vi "Memory.Pointer.Truncate U64.vi"(11 "U64":u64) -> (3 "truncated U64":u64)   [LabVIEW 2016, in "LabVIEW Memory Manager.lvlib" / "Memory.Pointer.lvclass"]
uses:
  Memory.Pointer.lvclass
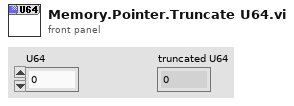
[diagram p1: front panel]
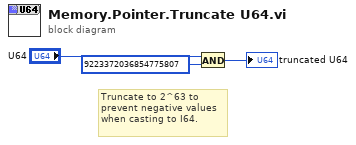
[diagram p0: block diagram]
diagram:
  # "Truncate to 2^63 to prevent negative values when casting to I64."
  n1 = And(x="U64", y=u64 9223372036854775807) -> (x .and. y?=→"truncated U64":u64)
